vi "Trav_pos_for_Email.vi"() -> (0 "String":string)   [LabVIEW 2017]
uses:
  Controls/Overhead.ctl
  Globals/Trav_pos_global.vi
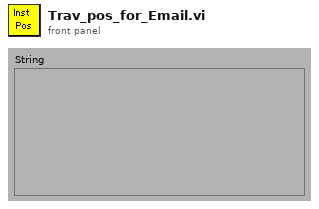
[diagram p1: front panel]
types:
  T1 = typedef "Overhead.ctl" = enum16{"Update total times", "Read Current Overhead", "Re Scale totals to 3 hrs", "Initialise totals to 3hr"}
  T2 = typedef "Tunnel_Coordinates.ctl" = enum16{"Work in Tunnel Coordinates", "Work in Model Coordinates"}
  T3 = typedef "Traverse_cluster.ctl" = cluster{"Start X":sgl, "Start Y":sgl, "Start Z":sgl, "End X":sgl, "End Y":sgl, "End Z":sgl, "No. of pts.":i32, "Spacing":T4, "Filename":path, "Tunnel Speed":dbl, "Averaging time (min)":dbl, "Extra Commands":string, "Carrier_1 Q (l/min)":dbl, "Carrier_2 Q (l/min)":dbl, "Trace Gas Concentration (%)":dbl, "Specific Arguments":string, "Comments":string, "Row No":i32, "Row Type Selector":T5, "Completion time":string, "Row Duration (mins)":dbl, "No. of Valid pts.":i32, "Meas Setup File":string}
  T4 = typedef "Spacing.ctl" = enum16{"Linear", "Log", "Gauss", "Specified", "N/A"}
  T5 = typedef "Multi_run_mode.ctl" = enum16{"Move Traverse Only", "Set Tunnel Speed Only", "Set Source Only", "Set Measurement Conditions", "Single Measurement", "Vertical Profile", "Lateral Profile", "Longitudinal Profile", "Explore Volume", "Multi-Axis Profile", "Auto Calibrate", "Meas Fast FID Bkgnd", "Check Beam Power", "Scanning Valve Measurement", "Run VI Named:", "Set ADAM Ch", "Wait (minutes)", "Send Message", "Synchronize With:", "Fall Back to this Row", "Turn Off Row Repeating", "Blank Row", "Traverse 3D Volume"}
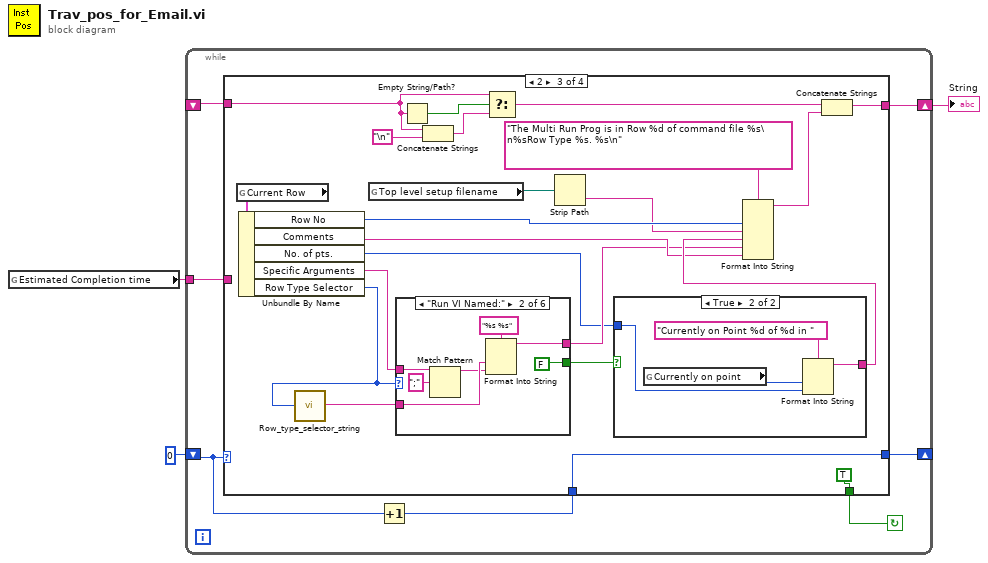
[diagram p0: block diagram]
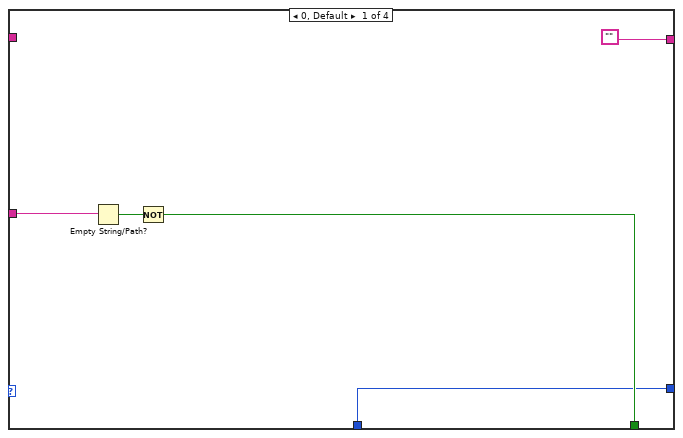
[diagram p2: hidden frame]
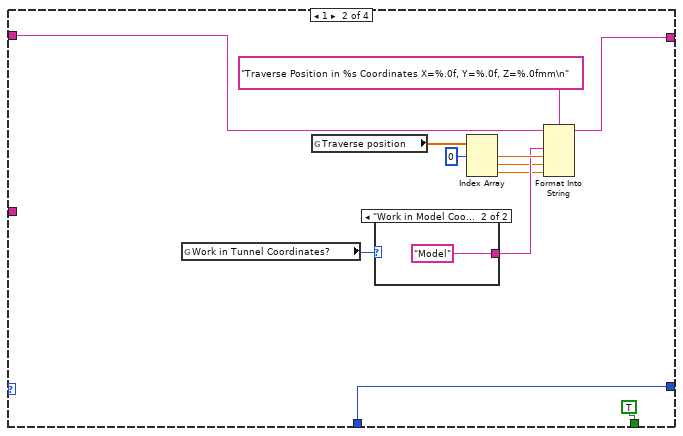
[diagram p3: hidden frame]
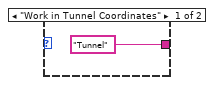
[diagram p4: hidden frame]
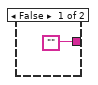
[diagram p5: hidden frame]
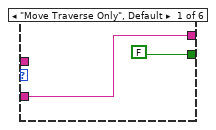
[diagram p6: hidden frame]
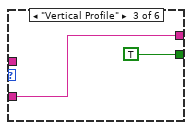
[diagram p7: hidden frame]
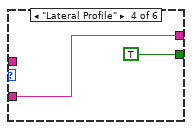
[diagram p8: hidden frame]
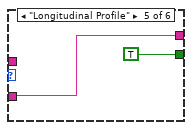
[diagram p9: hidden frame]
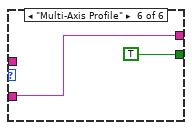
[diagram p10: hidden frame]
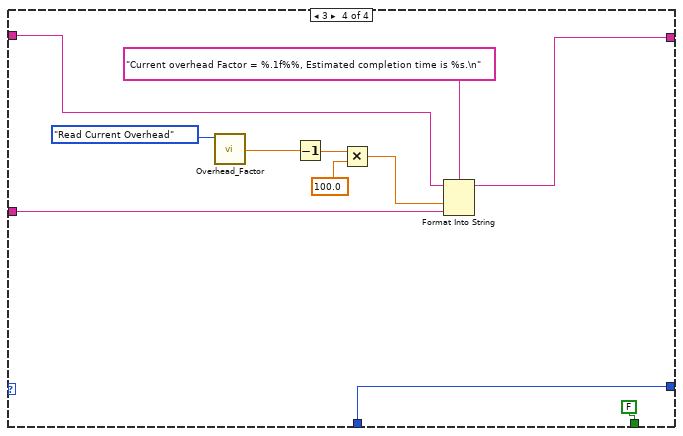
[diagram p11: hidden frame]
diagram:
  n1 = global read "Trav_pos_global.vi" "Estimated Completion time"() -> (w1:string)
  n2 = while {
    shift-left: _ -> [w5]
    shift-right: [w7] -> w2
    shift-left: 0 -> [w10]
    shift-right: [w9] -> _
    tunnel: w1 -> [w4]
    stop <- w6 continue-if-true
    n3 = Increment(x=w10) -> (x+1=w8:i32)
    n4 = case shown="2" w10 {
      tunnel: [w12 w27 w46 w83] -> w9
      tunnel: w8 -> [w12 w27 w46 w83]
      tunnel: ["" w22 w51 w75] -> w7
      tunnel: [w13 TRUE TRUE FALSE] -> w6
      tunnel: w5 -> [_ w23 w43 w76]
      tunnel: w4 -> [w15 _ _ w74]
      frame 0, Default {
        n5 = Empty String/Path?(string/path=w15) -> (empty?=w14:bool)
        n6 = Not(x=w14) -> (.not. x?=w13:bool)
      }
      frame 1 {
        n7 = global read "Trav_pos_global.vi" "Work in Tunnel Coordinates?"() -> (w21:T2)
        n8 = global read "Trav_pos_global.vi" "Traverse position"() -> (w18:sgl[])
        n9 = case shown="\"Work in Model Coordinates\"" w21 {
          tunnel: ["Tunnel" "Model"] -> w19
          frame "Work in Tunnel Coordinates" {
          }
          frame "Work in Model Coordinates" {
          }
        }
        n10 = Index Array(array=w18, index #1=0 ("index")) -> (element #1=w20:sgl, element #2=w17:sgl, element #3=w16:sgl)  [unwired: 2 in]
        n11 = Format Into String(format string="Traverse Position in %s Coordinates X=%.0f, Y=%.0f, Z=%.0fmm\n" ("Format String"), initial string=w23, w19, w20, w17, w16) -> (resulting string=w22:string)  [unwired: 1 in, 1 out]
      }
      frame 2 {
        n12 = global read "Trav_pos_global.vi" "Current Row"() -> (w38:T3)
        n13 = Unbundle By Name(w38) -> ("Row No"=w50:i32, "Comments"=w37:string, "No. of pts."=w32:i32, "Specific Arguments"=w34:string, "Row Type Selector"=w33:T5)
        n14 = call "Row_type_selector_string.vi"("Mode"=w33) -> ("Output string"=w36:string)
        n15 = global read "Trav_pos_global.vi" "Top level setup filename"() -> (w31:path)
        n16 = case shown="\"Run VI Named:\"" w33 {
          tunnel: [FALSE FALSE TRUE TRUE TRUE TRUE] -> w49
          tunnel: w36 -> [w57 w64 w66 w68 w70 w72]
          tunnel: [w57 w62 w66 w68 w70 w72] -> w35
          tunnel: w34 -> [_ w60 _ _ _ _]
          frame "Move Traverse Only", Default {
          }
          frame "Run VI Named:" {
            n17 = Match Pattern(string=w60, regular expression=";") -> (before substring=w59:string)  [unwired: 4 out]
            n18 = Format Into String(format string="%s %s" ("Format String"), w64, w59) -> (resulting string=w62:string)  [unwired: 2 in, 1 out]
          }
          frame "Vertical Profile" {
          }
          frame "Lateral Profile" {
          }
          frame "Longitudinal Profile" {
          }
          frame "Multi-Axis Profile" {
          }
        }
        n19 = Empty String/Path?(string/path=w43) -> (empty?=w45:bool)
        n20 = Concatenate Strings(w43, "\n") -> (w44:string)
        n21 = Select(t=w43, s=w45, f=w44) -> (s? t:f=w42:string)
        n22 = Strip Path(path=w31) -> (name=w30:string)  [unwired: 1 out]
        n23 = case shown="True" w49 {
          tunnel: w32 -> [_ w55]
          tunnel: ["" w53] -> w40
          frame False {
          }
          frame True {
            n24 = global read "Trav_pos_global.vi" "Currently on point"() -> (w56:i32)
            n25 = Format Into String(format string="Currently on Point %d of %d in " ("Format String"), w56, w55) -> (resulting string=w53:string)  [unwired: 2 in, 1 out]
          }
        }
        n26 = Format Into String(format string="The Multi Run Prog is in Row %d of command file %s\n%sRow Type %s. %s\n" ("Format String"), w50, w30, w40, w35, w37) -> (resulting string=w39:string)  [unwired: 2 in, 1 out]
        n27 = Concatenate Strings(w42, w39) -> (w51:string)
      }
      frame 3 {
        n28 = call "Overhead_Factor.vi"("Mode"=Overhead."Read Current Overhead") -> ("Current Overhead Factor"=w81:dbl)  [unwired: 3 in]
        n29 = Decrement(x=w81) -> (x-1=w80:dbl)
        n30 = Multiply(x=w80, y=100.0) -> (x*y=w78:dbl)
        n31 = Format Into String(format string="Current overhead Factor = %.1f%%, Estimated completion time is %s.\n" ("Format String"), initial string=w76, w78, w74) -> (resulting string=w75:string)  [unwired: 1 in, 1 out]
      }
    }
  }
  "String" <- w2
